vi "readout_convert (SubVI).vi"(1 "read buffer":string) -> (0 "Numeric":i32)   [LabVIEW 2013]
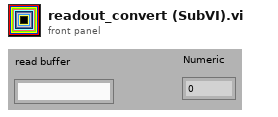
[diagram p1: front panel]
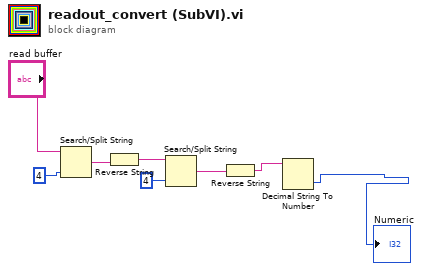
[diagram p0: block diagram]
diagram:
  n1 = Search/Split String(string="read buffer", offset (0)=4) -> (match + rest of string=w5:string)  [unwired: 1 in, 2 out]
  n2 = Reverse String(1:w5) -> (0:w4:string)
  n3 = Search/Split String(string=w4, offset (0)=4 ("offset (0) 2")) -> (match + rest of string=w3:string)  [unwired: 1 in, 2 out]
  n4 = Reverse String(1:w3) -> (0:w2:string)
  n5 = Decimal String To Number(string=w2) -> (number=→"Numeric":i32)  [unwired: 2 in, 1 out]
